vi "updateShipInfo.vi"(11 "template (empty)":path=path "O:/Monitor/回貨明細/temp/早車必回_0427.xls") -> ()   [LabVIEW 2012]
uses:
  <vilib>/Utility/NIReport.llb/NI_report.lvclass
  <vilib>/addons/database/Connection.llb/DB Tools Open Connec (Path).vi
  <vilib>/addons/_office/excel.llb/Excel Get Data (str).vi
  <vilib>/addons/_office/excel.llb/Excel Get Data (i32).vi
  <vilib>/addons/database/Connection.llb/Conn Execute.vi
  <vilib>/addons/database/Recordset.llb/Rec Fetch Integer Data (R).vi
  <vilib>/addons/database/Recordset.llb/Rec Destroy - Connection.vi
  <vilib>/Utility/NIReport.llb/Excel/NI_Excel.lvclass
  <vilib>/addons/_office/NI_ReportGenerationToolkit.lvlib
  <vilib>/addons/database/NI_Database_API.lvlib
panel:
  out "concatenated string 3":string
  out "concatenated string 2":string
  out "concatenated string":string
  out "error out":errorcluster
  out "data 2":string
  out "error out 4":errorcluster
  out "data":i32
  out "stime":i32
  out "sdate":i32
  out "Step":string
  out "Qty":i32
  out "Route":string
  out "Type":string
  in  "start (0, 0) 2":cluster{"start row":i32, "start column":i32}
  in  "start (0, 0)":cluster{"start row":i32, "start column":i32}
  out "row":i32
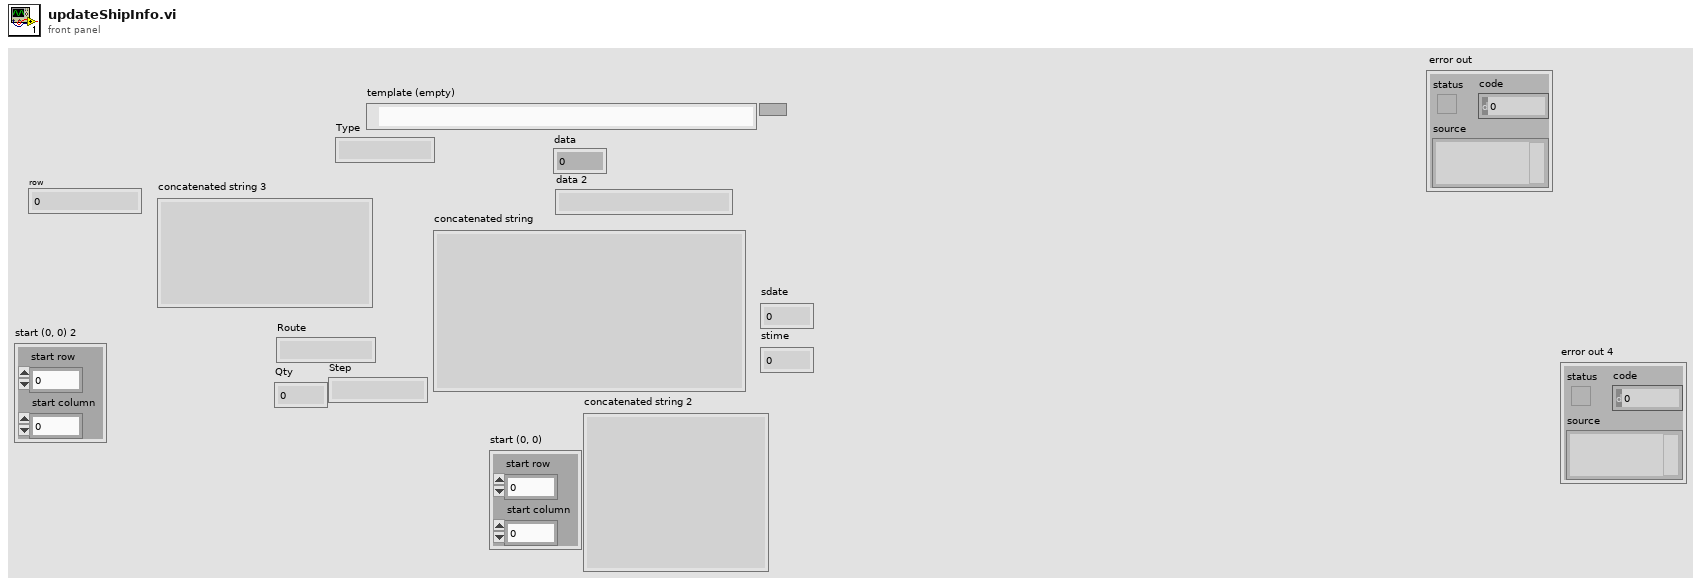
[diagram p1: front panel]
types:
  T1 = enum16{"Standard Report", "HTML", "Word", "Excel"}
  T2 = typedef "NI_Database_API.lvlib/Conn ObjectReference.ctl" = refnum<k1>
  T3 = typedef "NI_Database_API.lvlib/Rec ObjectReference.ctl" = refnum<k1>
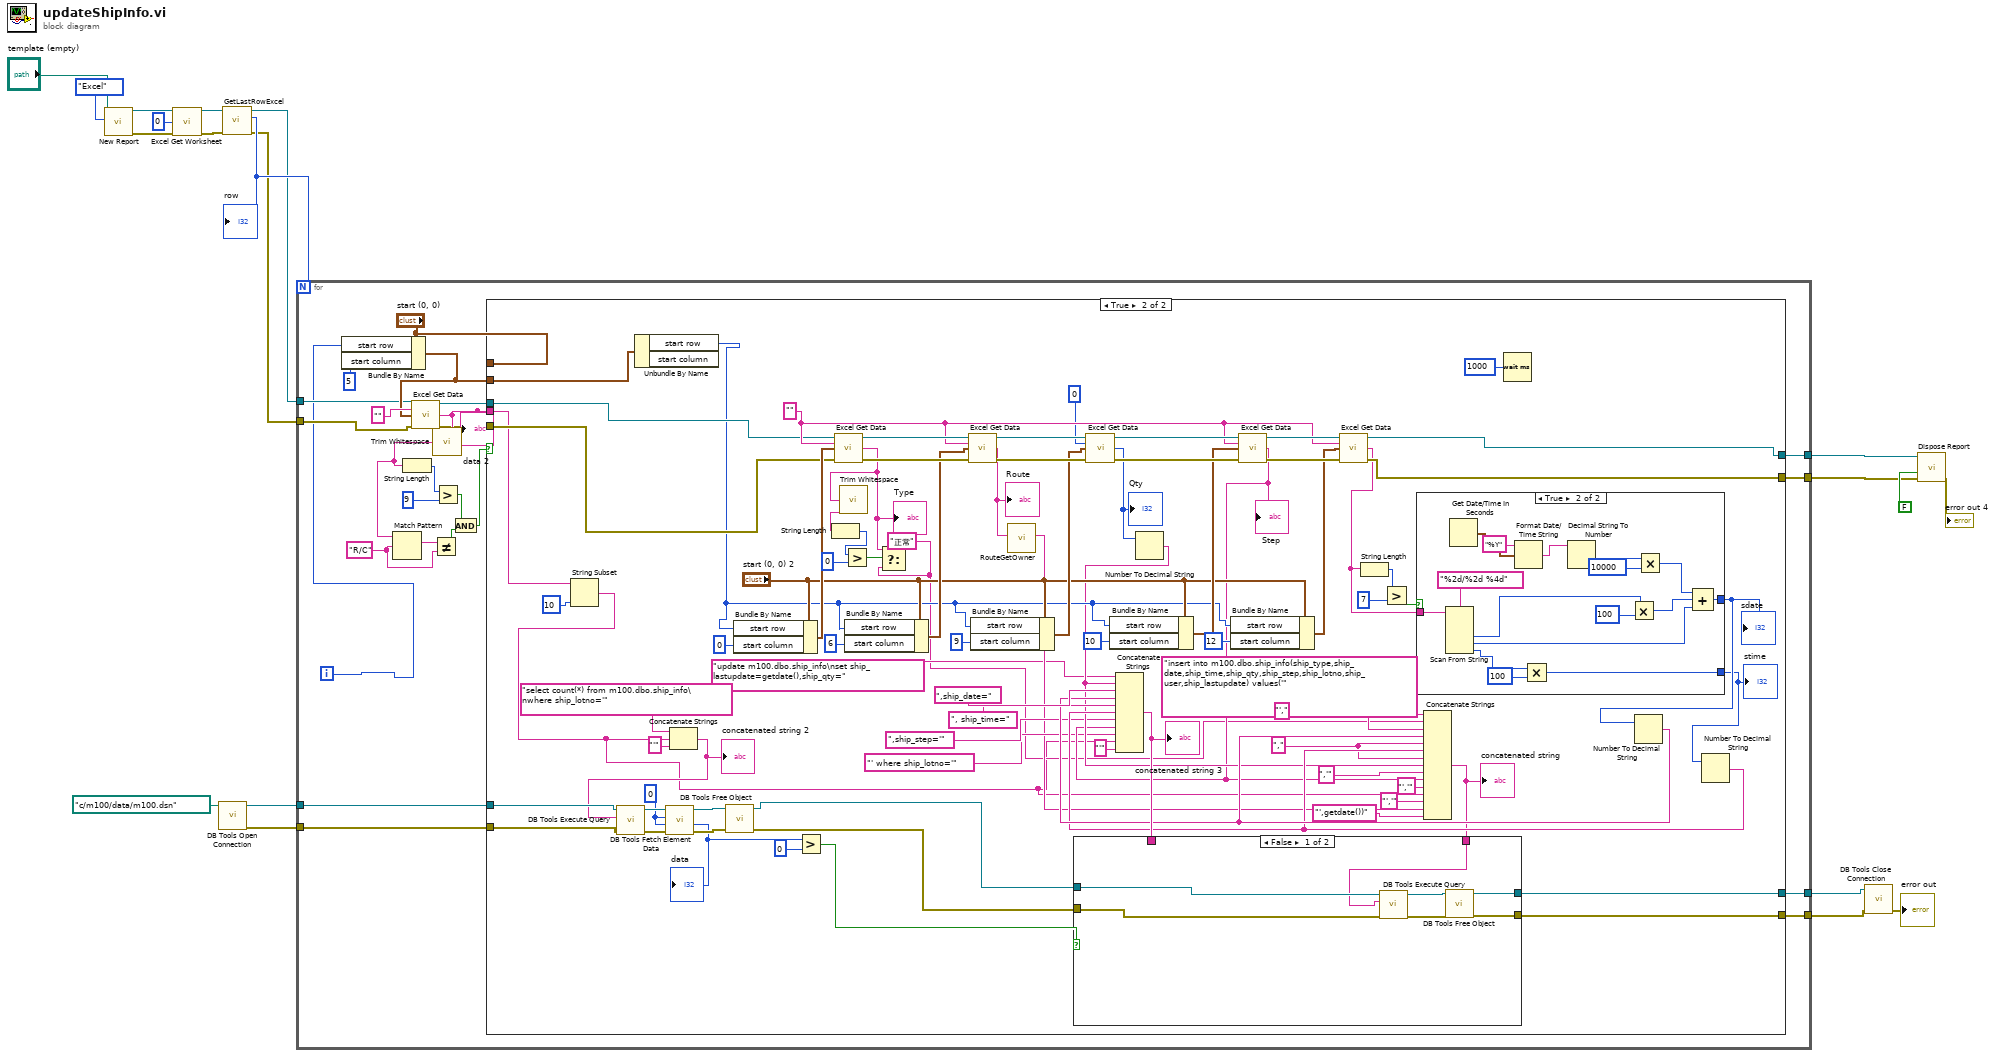
[diagram p0: block diagram]
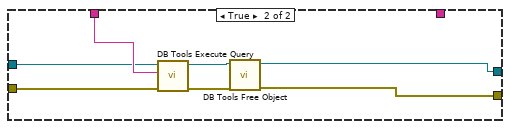
[diagram p3: hidden frame]
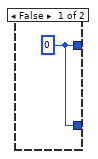
[diagram p4: hidden frame]
diagram:
  n1 = call <vilib>:"New Report.vi"("report type"=T1."Excel" ("Report Type"), "template (empty)"="template (empty)") -> ("report out"=w19:refnum<class "NI_report.lvclass">, "error out"=w18:errorcluster)  [unwired: 12 in]
  n2 = call <vilib>:"Excel Get Worksheet.vi"("report in"=w19, "worksheet index (0)"=0, "error in (no error)"=w18) -> ("report out"=w17:refnum<class "NI_report.lvclass">, "error out"=w16:errorcluster)  [unwired: 11 in]
  n3 = call-poly <vilib>:"DB Tools Open Connection.vi"("connection information"=path "c:/m100/data/m100.dsn") -> ("error out"=w9:errorcluster, "connection reference"=w10:T2)  [unwired: 7 in]
  n4 = call "GetLastRowExcel.vi"("error in (no error)"=w16, "report in"=w17) -> ("error out"=w12:errorcluster, "row"=w13:i32, "report out"=w11:refnum<class "NI_report.lvclass">)  [unwired: 7 in]
  "row" <- w13
  n5 = for {
    N: w13 -> [_]
    tunnel: w11 -> [w33]
    tunnel: w12 -> [w32]
    tunnel: [w36] -> w4
    tunnel: [w35] -> w3
    tunnel: w10 -> [w30]
    tunnel: w9 -> [w29]
    tunnel: [w28] -> w8
    tunnel: [w27] -> w7
    i -> [w31]
    w24 = "R/C" ("regular expression")
    n6 = Bundle By Name(cluster="start (0, 0)", "start row"=w31, "start column"=5) -> (w34:cluster{"start row":i32, "start column":i32})
    n7 = call-poly <vilib>:"Excel Get Data.vi"("report in"=w33, "data type"="", "start (0, 0)"=w34, "error in (no error)"=w32) -> ("report out"=w38:refnum<class "NI_report.lvclass">, "data"=w40:string, "error out"=w37:errorcluster)  [unwired: 9 in]
    "data 2" <- w40
    n8 = call <vilib>:"Trim Whitespace.vi"("string"=w40) -> ("trimmed string"=w26:string)  [unwired: 1 in]
    n9 = Match Pattern(string=w26, regular expression=w24) -> (match substring=w25:string)  [unwired: 1 in, 3 out]
    n10 = String Length(string=w26) -> (length=w41:i32)
    n11 = Not Equal?(x=w25, y=w24) -> (x != y?=w23:bool)
    n12 = Greater?(x=w41, y=9) -> (0:w22:bool)
    n13 = And(x=w22, y=w23) -> (x .and. y?=w21:bool)
    n14 = case shown="True" w21 {
      tunnel: w40 -> [_ w52]
      tunnel: "start (0, 0)" -> [_ _]
      tunnel: w38 -> [w48 w108]
      tunnel: w37 -> [w47 w107]
      tunnel: [w48 w55] -> w36
      tunnel: [w47 w105] -> w35
      tunnel: w34 -> [_ w130]
      tunnel: w30 -> [w46 w96]
      tunnel: w29 -> [w45 w95]
      tunnel: [w46 w66] -> w28
      tunnel: [w45 w65] -> w27
      frame False {
      }
      frame True {
        w53 = "正常" ("f")
        w75 = "," ("string")
        w91 = 0
        w110 = ""
        n15 = String Subset(string=w52, length (rest)=10 ("length (rest)")) -> (substring=w51:string)  [unwired: 1 in]
        n16 = Unbundle By Name(w130) -> ("start row"=w106:i32)  [unwired: 1 out]
        n17 = Concatenate Strings("select count(*) from m100.dbo.ship_info\nwhere ship_lotno='" ("string"), w51, "'" ("string")) -> (w92:string)
        "concatenated string 2" <- w92
        n18 = call-poly <vilib>:"DB Tools Execute Query.vi"("error in (no error)"=w95, "SQL query"=w92, "connection reference"=w96) -> ("error out"=w100:errorcluster, "recordset reference"=w99:T3)  [unwired: 5 in]
        n19 = call-poly <vilib>:"DB Tools Fetch Element Data.vi"("error in (no error)"=w100, "type"=w91, "column index"=w91, "recordset reference"=w99) -> ("error out"=w98:errorcluster, "data"=w90:i32, "recordset reference out"=w97:T3)  [unwired: 3 in]
        "data" <- w90
        n20 = call-poly <vilib>:"DB Tools Free Object.vi"("error in (no error)"=w98, "recordset reference"=w97) -> ("error out"=w80:errorcluster, "connection reference"=w81:T2)  [unwired: 8 in]
        n21 = Bundle By Name(cluster="start (0, 0) 2", "start row"=w106, "start column"=0) -> (w129:cluster{"start row":i32, "start column":i32})
        n22 = Greater?(x=w90, y=0) -> (0:w88:bool)
        n23 = call-poly <vilib>:"Excel Get Data.vi"("report in"=w108, "data type"=w110, "start (0, 0)"=w129, "error in (no error)"=w107) -> ("report out"=w127:refnum<class "NI_report.lvclass">, "data"=w56:string, "error out"=w126:errorcluster)  [unwired: 9 in]
        "Type" <- w56
        n24 = call <vilib>:"Trim Whitespace.vi"("string"=w56) -> ("trimmed string"=w60:string)  [unwired: 1 in]
        n25 = String Length(string=w60) -> (length=w59:i32)
        n26 = Greater?(x=w59, y=0) -> (0:w57:bool)
        n27 = Bundle By Name(cluster="start (0, 0) 2", "start row"=w106, "start column"=6) -> (w116:cluster{"start row":i32, "start column":i32})
        n28 = Select(t=w56, s=w57, f=w53) -> ()  [unwired: 1 out]
        n29 = call-poly <vilib>:"Excel Get Data.vi"("report in"=w127, "data type"=w110, "start (0, 0)"=w116, "error in (no error)"=w126) -> ("report out"=w125:refnum<class "NI_report.lvclass">, "data"=w64:string, "error out"=w124:errorcluster)  [unwired: 9 in]
        "Route" <- w64
        n30 = Bundle By Name(cluster="start (0, 0) 2", "start row"=w106, "start column"=9) -> (w117:cluster{"start row":i32, "start column":i32})
        n31 = call "RouteGetOwner.vi"("Route"=w64) -> ("Owner"=w61:string)  [unwired: 10 in]
        n32 = call-poly <vilib>:"Excel Get Data.vi"("report in"=w125, "data type"=0, "start (0, 0)"=w117, "error in (no error)"=w124) -> ("report out"=w123:refnum<class "NI_report.lvclass">, "data"=w87:i32, "error out"=w122:errorcluster)  [unwired: 9 in]
        "Qty" <- w87
        n33 = Bundle By Name(cluster="start (0, 0) 2", "start row"=w106, "start column"=10) -> (w118:cluster{"start row":i32, "start column":i32})
        n34 = Number To Decimal String(number=w87) -> (decimal integer string=w74:string)  [unwired: 1 in]
        n35 = Bundle By Name(cluster="start (0, 0) 2", "start row"=w106, "start column"=12) -> (w111:cluster{"start row":i32, "start column":i32})
        n36 = call-poly <vilib>:"Excel Get Data.vi"("report in"=w123, "data type"=w110, "start (0, 0)"=w118, "error in (no error)"=w122) -> ("report out"=w115:refnum<class "NI_report.lvclass">, "data"=w71:string, "error out"=w114:errorcluster)  [unwired: 9 in]
        "Step" <- w71
        n37 = call-poly <vilib>:"Excel Get Data.vi"("report in"=w115, "data type"=w110, "start (0, 0)"=w111, "error in (no error)"=w114) -> ("report out"=w55:refnum<class "NI_report.lvclass">, "data"=w101:string, "error out"=w105:errorcluster)  [unwired: 9 in]
        n38 = String Length(string=w101) -> (length=w104:i32)
        n39 = Greater?(x=w104, y=7) -> (0:w102:bool)
        n40 = case shown="True" w102 {
          tunnel: w101 -> [_ w148]
          tunnel: [w145 w147] -> w85
          tunnel: [w145 w146] -> w83
          frame False {
            w145 = 0
          }
          frame True {
            n41 = Scan From String(format string="%2d/%2d %4d", input string=w148) -> (output 1=w155:i32, output 2=w151:i32, output 3=w150:i32)  [unwired: 5 in, 3 out]
            n42 = Get Date/Time In Seconds() -> (seconds since 1Jan1904=w160:timestamp)
            n43 = Format Date/Time String(time format string (%c)="%Y", seconds (now)=w160) -> (date/time string=w158:string)  [unwired: 1 in]
            n44 = Multiply(x=w150, y=100) -> (x*y=w146:i32)
            n45 = Decimal String To Number(string=w158) -> (number=w157:i32)  [unwired: 2 in, 1 out]
            n46 = Multiply(x=w155, y=100) -> (x*y=w152:i32)
            n47 = Multiply(x=w157, y=10000) -> (x*y=w153:i32)
            n48 = Compound Arithmetic op=ADD(w153, w152, w151) -> (w147:i32)
          }
        }
        "sdate" <- w85
        "stime" <- w83
        n49 = Wait (ms)(milliseconds to wait=u32 1000) -> ()  [unwired: 1 out]
        n50 = Number To Decimal String(number=w85) -> (decimal integer string=w77:string)  [unwired: 1 in]
        n51 = Number To Decimal String(number=w83) -> (decimal integer string=w76:string)  [unwired: 1 in]
        n52 = Concatenate Strings("update m100.dbo.ship_info\nset ship_lastupdate=getdate(),ship_qty=" ("string"), w74, ",ship_date=" ("string"), w77, ", ship_time=" ("string"), w76, ",ship_step='" ("string"), w71, "' where ship_lotno='" ("string"), w51, "'" ("string")) -> (w82:string)
        "concatenated string 3" <- w82
        n53 = Concatenate Strings("insert into m100.dbo.ship_info(ship_type,ship_date,ship_time,ship_qty,ship_step,ship_lotno,ship_user,ship_lastupdate) values('" ("string"), w53, "'," ("string"), w77, w75, w76, w75, w74, ",'" ("string"), w71, "','" ("string"), w51, "','" ("string"), w61, "',getdate())" ("string")) -> (w68:string)
        "concatenated string" <- w68
        n54 = case shown="False" w88 {
          tunnel: w82 -> [_ w144]
          tunnel: w81 -> [w135 w143]
          tunnel: w80 -> [w134 w142]
          tunnel: w68 -> [w133 _]
          tunnel: [w132 w139] -> w66
          tunnel: [w131 w138] -> w65
          frame False {
            n55 = call-poly <vilib>:"DB Tools Execute Query.vi"("error in (no error)"=w134, "SQL query"=w133, "connection reference"=w135) -> ("error out"=w137:errorcluster, "recordset reference"=w136:T3)  [unwired: 5 in]
            n56 = call-poly <vilib>:"DB Tools Free Object.vi"("error in (no error)"=w137, "recordset reference"=w136) -> ("error out"=w131:errorcluster, "connection reference"=w132:T2)  [unwired: 8 in]
          }
          frame True {
            n57 = call-poly <vilib>:"DB Tools Execute Query.vi"("error in (no error)"=w142, "SQL query"=w144, "connection reference"=w143) -> ("error out"=w140:errorcluster, "recordset reference"=w141:T3)  [unwired: 5 in]
            n58 = call-poly <vilib>:"DB Tools Free Object.vi"("error in (no error)"=w140, "recordset reference"=w141) -> ("error out"=w138:errorcluster, "connection reference"=w139:T2)  [unwired: 8 in]
          }
        }
      }
    }
  }
  n59 = call <vilib>:"DB Tools Close Connection.vi"("error in (no error)"=w7, "connection reference"=w8) -> ("error out"=→"error out":errorcluster)  [unwired: 5 in]
  n60 = call-dynamic "Dispose Report.vi"("report in"=w4, "save changes? (F)"=FALSE, "error in (no error)"=w3) -> ("error out"=→"error out 4":errorcluster)  [unwired: 12 in]
